vi "subImage_UpdateBin.vi"(4 "Bin (n x n)":u16(ring)=4 items=["1x1"=1, "2x2"=2, "4x4"=4], 6 "Previous bin":u16(ring)=1 caption="Previous Bin" items=["1x1"=1, "2x2"=2, "4x4"=4], 7 "Image Refnum":refnum<vi>, 11 "ROI in":T1={"Bin"=4, "ROI"={"x offset"=0, "y offset"=0, "x width"=512, "y width"=512}} {"ROI"."x offset" min=1 max=512 step=1; "ROI"."y offset" min=1 max=512 step=1; "ROI"."x width" min=1 max=512 step=1; "ROI"."y width" min=1 max=512 step=1; "Bin" items=["1x1"=1, "2x2"=2, "4x4"=4]}) -> (3 "ROI out":T1={"Bin"=4, "ROI"={"x offset"=0, "y offset"=0, "x width"=512, "y width"=512}} {"ROI"."x offset" min=1 max=512 step=1; "ROI"."y offset" min=1 max=512 step=1; "ROI"."x width" min=1 max=512 step=1; "ROI"."y width" min=1 max=512 step=1; "Bin" items=["1x1"=1, "2x2"=2, "4x4"=4]})   [LabVIEW 2015]
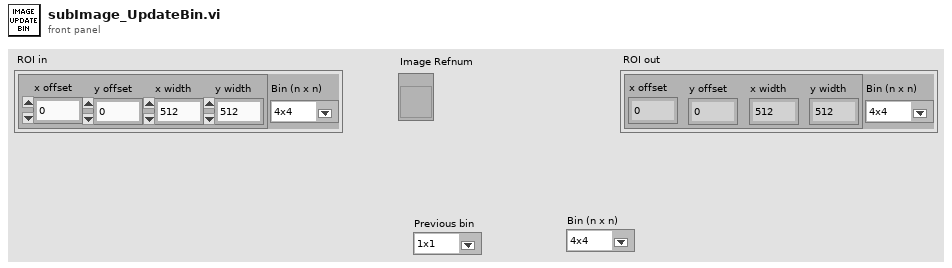
[diagram p1: front panel]
types:
  T1 = cluster{"Bin":u16, "ROI":cluster{"x offset":i32, "y offset":i32, "x width":i32, "y width":i32}}
  T2 = typedef "LVPointDoubleTypeDef.ctl" = cluster{"Cursor X":dbl, "Cursor Y":dbl}
  T3 = cluster{"x offset":i32, "y offset":i32, "x width":i32, "y width":i32}
  T4 = cluster{"Cursor.Cursor Position":T2, "Cursor.Cursor Position":T2, "XScale.Minimum":dbl, "YScale.Minimum":dbl, "XScale.Maximum":dbl, "YScale.Maximum":dbl, "ROI":cluster{"x offset":i32, "y offset":i32, "x width":i32, "y width":i32}}
  T5 = cluster{"Cursor.Cursor Position":T2, "Cursor.Cursor Position":T2, "XScale.Minimum":dbl, "YScale.Minimum":dbl, "XScale.Maximum":dbl, "YScale.Maximum":dbl, "ROI":cluster{"x offset":dbl, "y offset":dbl, "x width":dbl, "y width":dbl}}
  T6 = cluster{"x offset":dbl, "y offset":dbl, "x width":dbl, "y width":dbl}
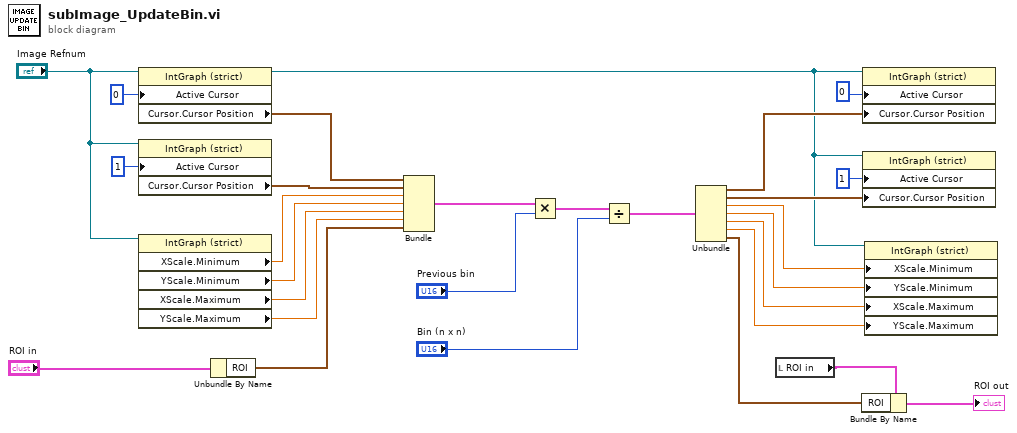
[diagram p0: block diagram]
diagram:
  n1 = property on="Property Node" class="IntGraph (strict)"(reference="Image Refnum", "Active Cursor"=u32 0) -> (reference out=w3:refnum<vi>, "Cursor.Cursor Position"=w22:T2)  [unwired: 1 in, 1 out]
  n2 = property on="Property Node" class="IntGraph (strict)"(reference="Image Refnum", "Active Cursor"=u32 1) -> ("Cursor.Cursor Position"=w21:T2)  [unwired: 1 in, 2 out]
  n3 = property on="Property Node" class="IntGraph (strict)"(reference="Image Refnum") -> ("XScale.Minimum"=w20:dbl, "YScale.Minimum"=w19:dbl, "XScale.Maximum"=w18:dbl, "YScale.Maximum"=w17:dbl)  [unwired: 1 in, 2 out]
  n4 = Unbundle By Name("ROI in") -> ("ROI"=w7:T3)
  n5 = Bundle("Cursor.Cursor Position"=w22, "Cursor.Cursor Position"=w21, "XScale.Minimum"=w20, "YScale.Minimum"=w19, "XScale.Maximum"=w18, "YScale.Maximum"=w17, "ROI"=w7) -> (w16:T4)  [unwired: 1 in]
  n6 = Multiply(x=w16, y="Previous bin") -> (x*y=w23:T4)
  n7 = Divide(x=w23, y="Bin (n x n)") -> (x/y=w15:T5)
  n8 = Unbundle(w15) -> ("Cursor.Cursor Position"=w14:T2, "Cursor.Cursor Position"=w13:T2, "XScale.Minimum"=w12:dbl, "YScale.Minimum"=w11:dbl, "XScale.Maximum"=w10:dbl, "YScale.Maximum"=w9:dbl, "ROI"=w6:T6)
  n9 = local read "ROI in"() -> (w1:T1)
  n10 = Bundle By Name(cluster=w1, "ROI"=w6) -> (→"ROI out":T1)
  n11 = property on="Property Node" class="IntGraph (strict)"(reference=w3, "Active Cursor"=u32 0, "Cursor.Cursor Position"=w14) -> ()  [unwired: 1 in, 2 out]
  n12 = property on="Property Node" class="IntGraph (strict)"(reference=w3, "Active Cursor"=u32 1, "Cursor.Cursor Position"=w13) -> ()  [unwired: 1 in, 2 out]
  n13 = property on="Property Node" class="IntGraph (strict)"(reference=w3, "XScale.Minimum"=w12, "YScale.Minimum"=w11, "XScale.Maximum"=w10, "YScale.Maximum"=w9) -> ()  [unwired: 1 in, 2 out]
